vi "Configure Waveforms.vi"(8 "error in (no error)":errorcluster, 10 "Waveform paths":string[](array[string]), 11 "Gateway IP Address (\"\": localhost)":string) -> (0 "error out":errorcluster, 1 "waveform data event registration (DBL)":refnum<event-registration>, 2 "WaveformStreamSpecifications":T1[](array[typedef]), 3 "WaveformStreaming out":T2)   [LabVIEW 2015]
uses:
  <vilib>/NI Veristand/Execution/WaveformStreaming/Waveform Data Watcher Event Data (DBL).ctl
  <vilib>/NI Veristand/Execution/WaveformStreaming/WaveformStreamSpecification.ctl
  NationalInstruments.VeriStand.ClientAPI
  <vilib>/NI Veristand/Execution/WaveformStreaming/WaveformStreamingAPI.ctl
  <vilib>/NI Veristand/Execution/WaveformStreaming/Set Rate for Waveform Stream (Acquisition Rate).vi
  <vilib>/NI Veristand/Execution/WaveformStreaming/Set Condition for Waveform Stream (All Data).vi
  <vilib>/NI Veristand/Execution/WaveformStreaming/Register for Waveform Data Events (DBL).vi
  <vilib>/NI Veristand/Execution/WaveformStreaming/NI_VS Waveform Streaming Interface.lvlib
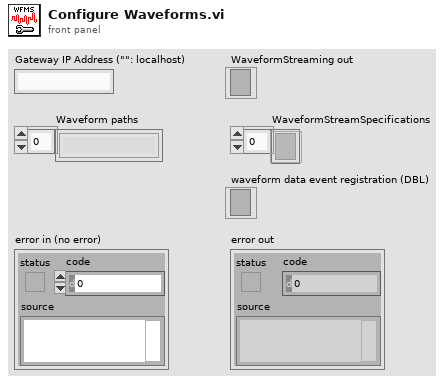
[diagram p1: front panel]
types:
  T1 = typedef "NI_VS Waveform Streaming Interface.lvlib/WaveformStreamSpecification.ctl" = refnum<k24>
  T2 = typedef "NI_VS Waveform Streaming Interface.lvlib/WaveformStreamingAPI.ctl" = refnum<k24>
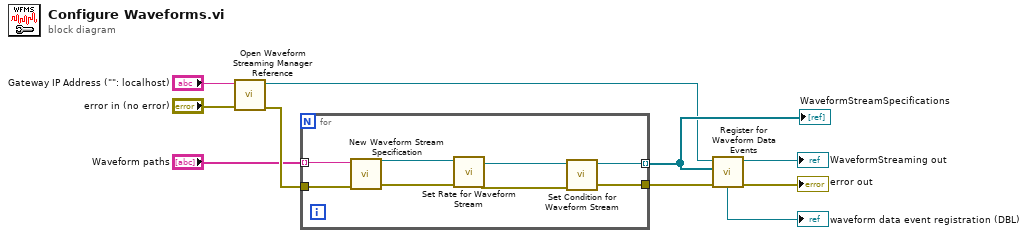
[diagram p0: block diagram]
diagram:
  n1 = call <vilib>:"Open Waveform Streaming Manager Reference.vi"("error in (no error)"="error in (no error)", "Gateway IP Address (\"\": localhost)"="Gateway IP Address (\"\": localhost)") -> ("error out"=w10:errorcluster, "WaveformStreaming"=w7:T2)  [unwired: 8 in]
  n2 = for {
    tunnel: "Waveform paths" -> [w18] mode=indexing
    tunnel: w10 -> [w17]
    tunnel: [w11] -> w8
    tunnel: [w12] -> w9 mode=indexing
    n3 = call <vilib>:"New Waveform Stream Specification.vi"("error in (no error)"=w17, "waveform path"=w18) -> ("error out"=w16:errorcluster, "WaveformStreamSpecification"=w15:T1)  [unwired: 8 in]
    n4 = call-poly <vilib>:"Set Rate for Waveform Stream.vi"("error in (no error)"=w16, "WaveformStreamSpecification in"=w15) -> ("error out"=w14:errorcluster, "WaveformStreamSpecification out"=w13:T1)  [unwired: 8 in]
    n5 = call-poly <vilib>:"Set Condition for Waveform Stream.vi"("error in (no error)"=w14, "WaveformStreamSpecification in"=w13) -> ("error out"=w11:errorcluster, "WaveformStreamSpecification out"=w12:T1)  [unwired: 8 in]
  }
  "WaveformStreamSpecifications" <- w9
  n6 = call-poly <vilib>:"Register for Waveform Data Events.vi"("error in (no error)"=w8, "WaveformStreamSpecifications"=w9, "WaveformStreaming in"=w7) -> ("error out"=→"error out":errorcluster, "WaveformStreaming out"=→"WaveformStreaming out":T2, "waveform data event registration (DBL)"=→"waveform data event registration (DBL)":refnum<event-registration>)  [unwired: 5 in, 1 out]
